vi "UIinit_setting.vi"(9 "Language":u32, 10 "VIref":refnum<vi>) -> ()   [LabVIEW 2015]
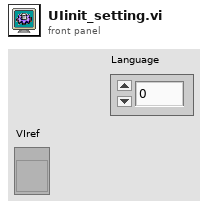
[diagram p1: front panel]
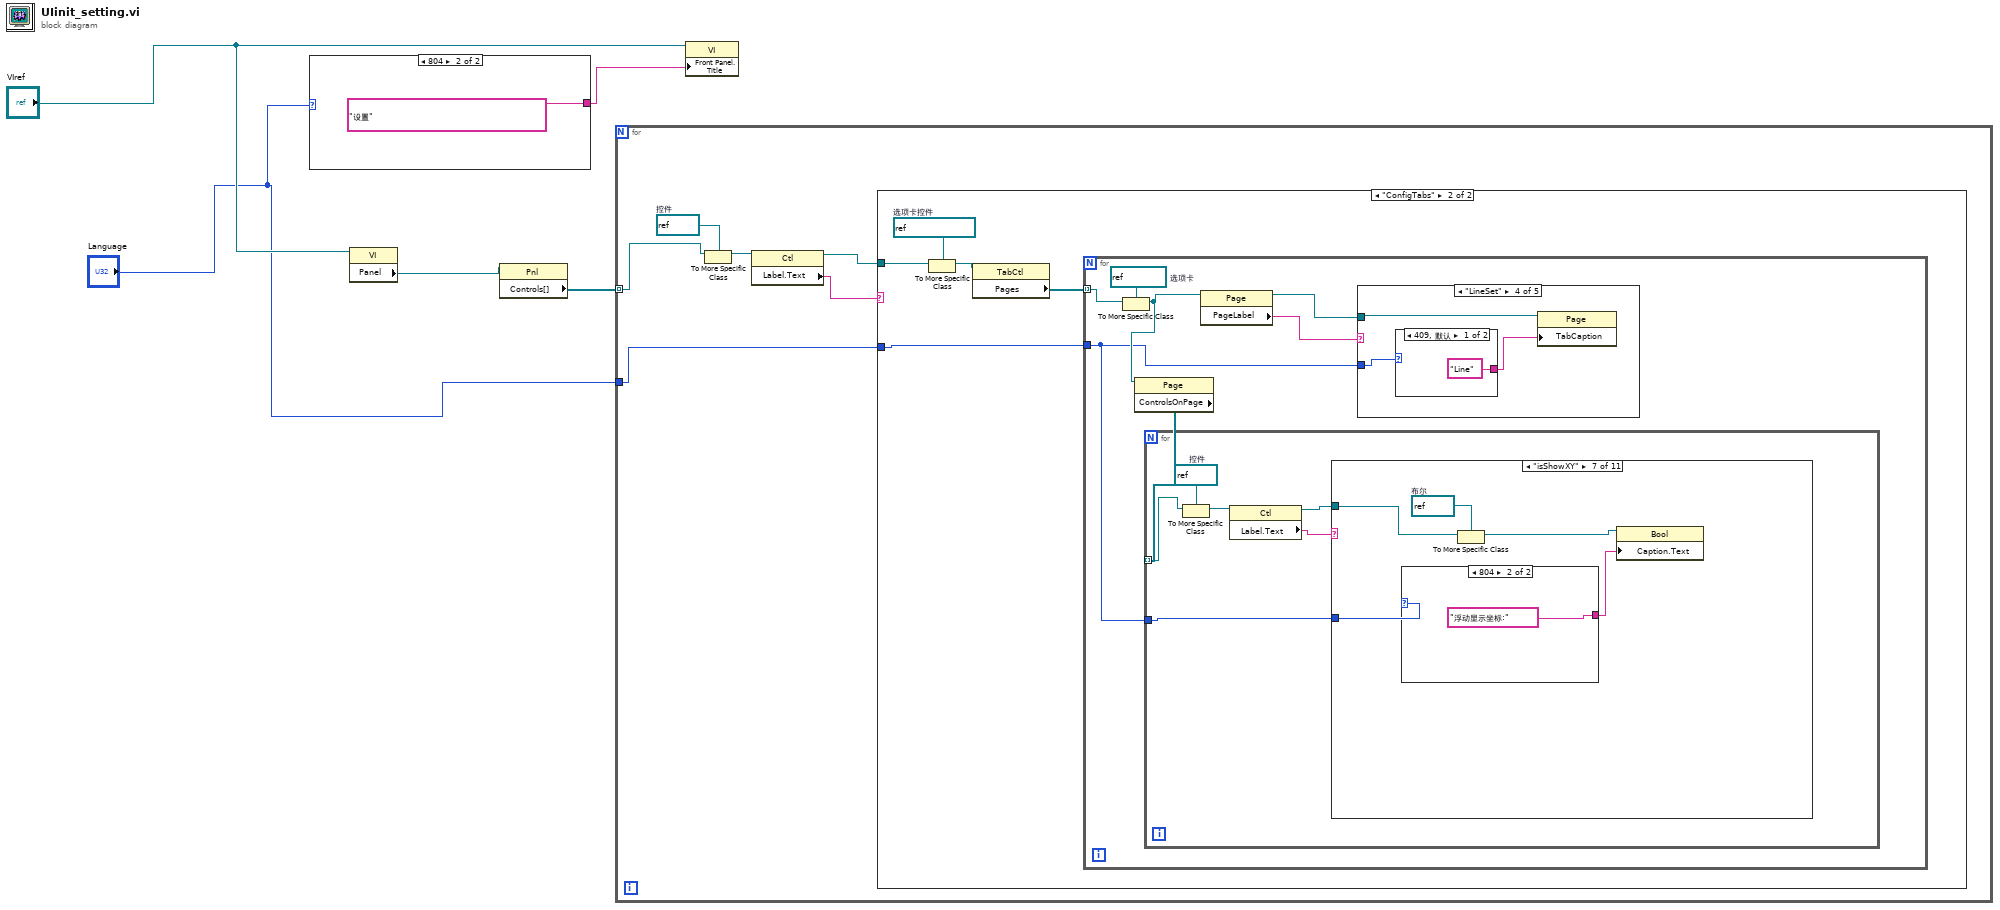
[diagram p0: block diagram]
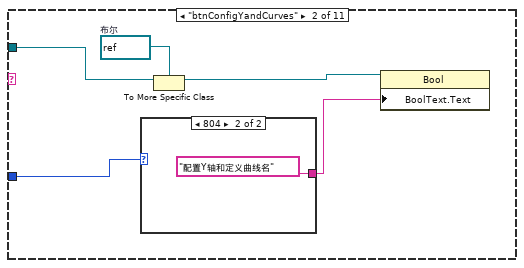
[diagram p4: hidden frame]
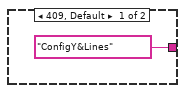
[diagram p5: hidden frame]
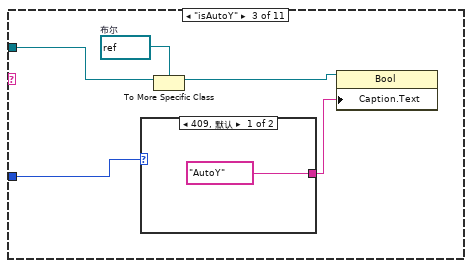
[diagram p6: hidden frame]
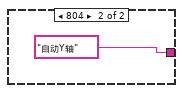
[diagram p7: hidden frame]
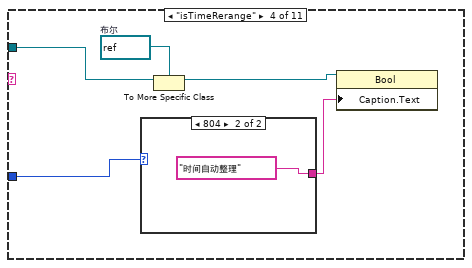
[diagram p8: hidden frame]
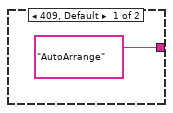
[diagram p9: hidden frame]
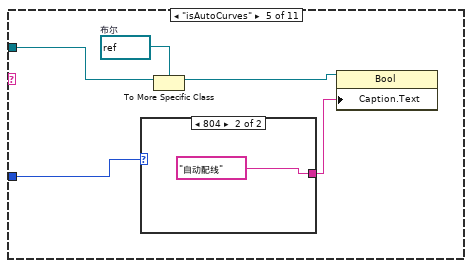
[diagram p10: hidden frame]
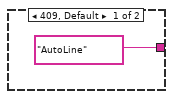
[diagram p11: hidden frame]
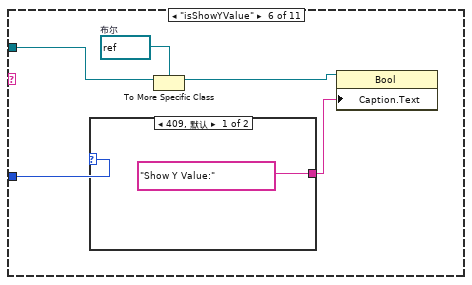
[diagram p12: hidden frame]
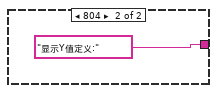
[diagram p13: hidden frame]
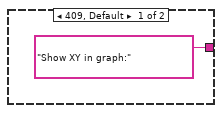
[diagram p14: hidden frame]
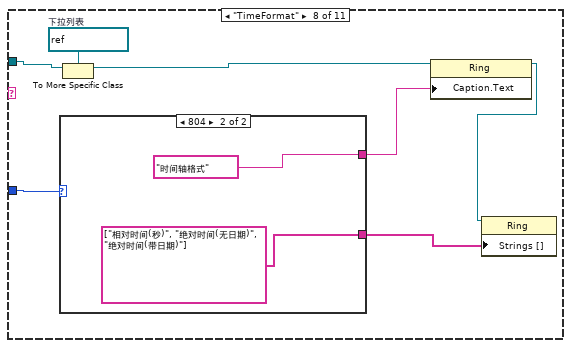
[diagram p15: hidden frame]
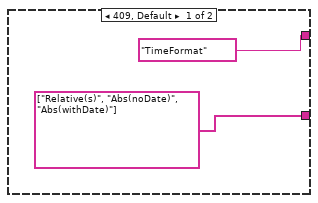
[diagram p16: hidden frame]
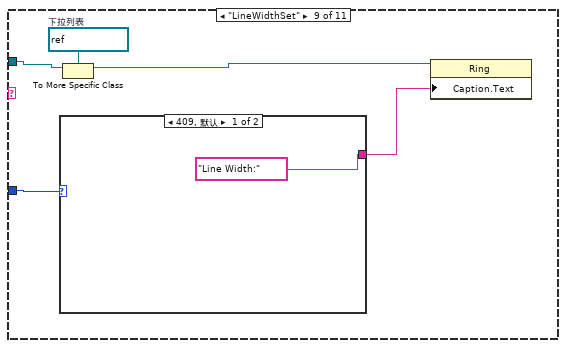
[diagram p17: hidden frame]
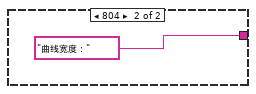
[diagram p18: hidden frame]
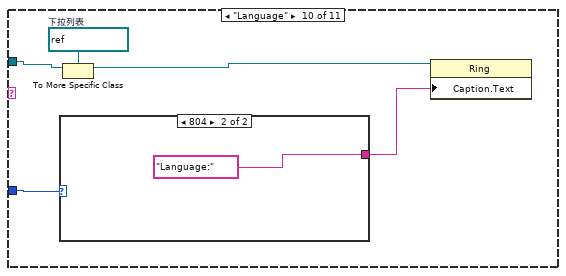
[diagram p19: hidden frame]
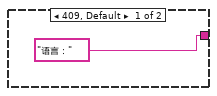
[diagram p20: hidden frame]
diagram:
  n1 = case shown="804" "Language" {
    tunnel: ["Settings" "设置"] -> w5
    frame 409, Default {
    }
    frame 804 {
    }
  }
  n2 = property class="VI"(reference="VIref") -> ("Panel"=w2:refnum<vi>)  [unwired: 1 in, 2 out]
  n3 = property class="Pnl"(reference=w2) -> ("Controls[]"=w3:refnum<vi>[])  [unwired: 1 in, 2 out]
  n4 = for {
    tunnel: w3 -> [w8] mode=indexing
    tunnel: "Language" -> [w9]
    w13 = refnum<vi> refnum  # 控件
    n5 = To More Specific Class(target class=w13, reference=w8) -> (specific class reference=w12:refnum<vi>)  [unwired: 1 in, 1 out]
    n6 = property class="Ctl"(reference=w12) -> (reference out=w10:refnum<vi>, "Label.Text"=w11:string)  [unwired: 1 in, 1 out]
    n7 = case shown="\"ConfigTabs\"" w11 {
      tunnel: w10 -> [_ w18]
      tunnel: w9 -> [_ w14]
      frame "假", Default {
      }
      frame "ConfigTabs" {
        w17 = refnum<vi> refnum  # 选项卡控件
        n8 = To More Specific Class(target class=w17, reference=w18) -> (specific class reference=w16:refnum<vi>)  [unwired: 1 in, 1 out]
        n9 = property class="TabCtl"(reference=w16) -> ("Pages"=w15:refnum<vi>[])  [unwired: 1 in, 2 out]
        n10 = for {
          tunnel: w15 -> [w22] mode=indexing
          tunnel: w14 -> [w19]
          w23 = refnum<vi> refnum  # 选项卡
          n11 = To More Specific Class(target class=w23, reference=w22) -> (specific class reference=w20:refnum<vi>)  [unwired: 1 in, 1 out]
          n12 = property class="Page"(reference=w20) -> ("ControlsOnPage"=w21:refnum<vi>[])  [unwired: 1 in, 2 out]
          n13 = for {
            tunnel: w21 -> [w26] mode=indexing
            tunnel: w19 -> [w27]
            w31 = refnum<vi> refnum  # 控件
            n14 = To More Specific Class(target class=w31, reference=w26) -> (specific class reference=w30:refnum<vi>)  [unwired: 1 in, 1 out]
            n15 = property class="Ctl"(reference=w30) -> (reference out=w28:refnum<vi>, "Label.Text"=w29:string)  [unwired: 1 in, 1 out]
            n16 = case shown="\"isShowXY\"" w29 {
              tunnel: w28 -> [_ w35 w42 w49 w56 w63 w70 w79 w88 w95 w104]
              tunnel: w27 -> [_ w36 w43 w50 w57 w64 w71 w78 w87 w94 w103]
              frame "假", Default {
              }
              frame "btnConfigYandCurves" {
                w34 = refnum<vi> refnum  # 布尔
                n17 = case shown="804" w36 {
                  tunnel: ["ConfigY&Lines" "配置Y轴和定义曲线名"] -> w32
                  frame 409, Default {
                  }
                  frame 804 {
                  }
                }
                n18 = To More Specific Class(target class=w34, reference=w35) -> (specific class reference=w33:refnum<vi>)  [unwired: 1 in, 1 out]
                n19 = property class="Bool"(reference=w33, "BoolText.Text"=w32) -> ()  [unwired: 1 in, 2 out]
              }
              frame "isAutoY" {
                w41 = refnum<vi> refnum  # 布尔
                n20 = case shown="409, 默认" w43 {
                  tunnel: ["AutoY" "自动Y轴"] -> w39
                  frame 409, Default {
                  }
                  frame 804 {
                  }
                }
                n21 = To More Specific Class(target class=w41, reference=w42) -> (specific class reference=w40:refnum<vi>)  [unwired: 1 in, 1 out]
                n22 = property class="Bool"(reference=w40, "Caption.Text"=w39) -> ()  [unwired: 1 in, 2 out]
              }
              frame "isTimeRerange" {
                w48 = refnum<vi> refnum  # 布尔
                n23 = case shown="804" w50 {
                  tunnel: ["AutoArrange" "时间自动整理"] -> w46
                  frame 409, Default {
                  }
                  frame 804 {
                  }
                }
                n24 = To More Specific Class(target class=w48, reference=w49) -> (specific class reference=w47:refnum<vi>)  [unwired: 1 in, 1 out]
                n25 = property class="Bool"(reference=w47, "Caption.Text"=w46) -> ()  [unwired: 1 in, 2 out]
              }
              frame "isAutoCurves" {
                w55 = refnum<vi> refnum  # 布尔
                n26 = case shown="804" w57 {
                  tunnel: ["AutoLine" "自动配线"] -> w53
                  frame 409, Default {
                  }
                  frame 804 {
                  }
                }
                n27 = To More Specific Class(target class=w55, reference=w56) -> (specific class reference=w54:refnum<vi>)  [unwired: 1 in, 1 out]
                n28 = property class="Bool"(reference=w54, "Caption.Text"=w53) -> ()  [unwired: 1 in, 2 out]
              }
              frame "isShowYValue" {
                w62 = refnum<vi> refnum  # 布尔
                n29 = case shown="409, 默认" w64 {
                  tunnel: ["Show Y Value:" "显示Y值定义:"] -> w60
                  frame 409, Default {
                  }
                  frame 804 {
                  }
                }
                n30 = To More Specific Class(target class=w62, reference=w63) -> (specific class reference=w61:refnum<vi>)  [unwired: 1 in, 1 out]
                n31 = property class="Bool"(reference=w61, "Caption.Text"=w60) -> ()  [unwired: 1 in, 2 out]
              }
              frame "isShowXY" {
                w69 = refnum<vi> refnum  # 布尔
                n32 = case shown="804" w71 {
                  tunnel: ["Show XY in graph:" "浮动显示坐标:"] -> w67
                  frame 409, Default {
                  }
                  frame 804 {
                  }
                }
                n33 = To More Specific Class(target class=w69, reference=w70) -> (specific class reference=w68:refnum<vi>)  [unwired: 1 in, 1 out]
                n34 = property class="Bool"(reference=w68, "Caption.Text"=w67) -> ()  [unwired: 1 in, 2 out]
              }
              frame "TimeFormat" {
                w80 = refnum<vi> refnum  # 下拉列表
                n35 = case shown="804" w78 {
                  tunnel: [string[] ["Relative(s)", "Abs(noDate)", "Abs(withDate)"] string[] ["相对时间(秒)", "绝对时间(无日期)", "绝对时间(带日期)"]] -> w77
                  tunnel: ["TimeFormat" "时间轴格式"] -> w74
                  frame 409, Default {
                  }
                  frame 804 {
                  }
                }
                n36 = To More Specific Class(target class=w80, reference=w79) -> (specific class reference=w76:refnum<vi>)  [unwired: 1 in, 1 out]
                n37 = property class="Ring"(reference=w76, "Caption.Text"=w74) -> (reference out=w75:refnum<vi>)  [unwired: 1 in, 1 out]
                n38 = property class="Ring"(reference=w75, "Strings []"=w77) -> ()  [unwired: 1 in, 2 out]
              }
              frame "LineWidthSet" {
                w89 = refnum<vi> refnum  # 下拉列表
                n39 = case shown="409, 默认" w87 {
                  tunnel: ["Line Width:" "曲线宽度："] -> w85
                  frame 409, Default {
                  }
                  frame 804 {
                  }
                }
                n40 = To More Specific Class(target class=w89, reference=w88) -> (specific class reference=w86:refnum<vi>)  [unwired: 1 in, 1 out]
                n41 = property class="Ring"(reference=w86, "Caption.Text"=w85) -> ()  [unwired: 1 in, 2 out]
              }
              frame "Language" {
                w96 = refnum<vi> refnum  # 下拉列表
                n42 = case shown="804" w94 {
                  tunnel: ["语言：" "Language:"] -> w92
                  frame 409, Default {
                  }
                  frame 804 {
                  }
                }
                n43 = To More Specific Class(target class=w96, reference=w95) -> (specific class reference=w93:refnum<vi>)  [unwired: 1 in, 1 out]
                n44 = property class="Ring"(reference=w93, "Caption.Text"=w92) -> ()  [unwired: 1 in, 2 out]
              }
              frame "ChkUpdatePeriod" {
                w105 = refnum<vi> refnum  # 下拉列表
                n45 = case shown="409, 默认" w103 {
                  tunnel: ["Check for updates:" "检查更新周期:"] -> w101
                  tunnel: [string[] ["EveryMonth", "EveryWeek", "Everyday", "EveryHour", "EveryRunning", "Never"] string[] ["每个月", "每星期", "每一天", "每小时", "每次运行", "从不"]] -> w99
                  frame 409, Default {
                  }
                  frame 804 {
                  }
                }
                n46 = To More Specific Class(target class=w105, reference=w104) -> (specific class reference=w102:refnum<vi>)  [unwired: 1 in, 1 out]
                n47 = property class="Ring"(reference=w102, "Caption.Text"=w101) -> (reference out=w100:refnum<vi>)  [unwired: 1 in, 1 out]
                n48 = property class="Ring"(reference=w100, "Strings []"=w99) -> ()  [unwired: 1 in, 2 out]
              }
            }
          }
          n49 = property class="Page"(reference=w20) -> (reference out=w24:refnum<vi>, "PageLabel"=w25:string)  [unwired: 1 in, 1 out]
          n50 = case shown="\"LineSet\"" w25 {
            tunnel: w19 -> [_ w112 w117 w122 w127]
            tunnel: w24 -> [_ w111 w116 w121 w126]
            frame "假", Default {
            }
            frame "Xset" {
              n51 = case shown="804" w112 {
                tunnel: ["X axis" "X轴"] -> w110
                frame 409, Default {
                }
                frame 804 {
                }
              }
              n52 = property class="Page"(reference=w111, "TabCaption"=w110) -> ()  [unwired: 1 in, 2 out]
            }
            frame "Yset" {
              n53 = case shown="804" w117 {
                tunnel: ["Y axis" "Y轴"] -> w115
                frame 409, Default {
                }
                frame 804 {
                }
              }
              n54 = property class="Page"(reference=w116, "TabCaption"=w115) -> ()  [unwired: 1 in, 2 out]
            }
            frame "LineSet" {
              n55 = case shown="409, 默认" w122 {
                tunnel: ["Line" "曲线"] -> w120
                frame 409, Default {
                }
                frame 804 {
                }
              }
              n56 = property class="Page"(reference=w121, "TabCaption"=w120) -> ()  [unwired: 1 in, 2 out]
            }
            frame "UI" {
              n57 = case shown="409, 默认" w127 {
                tunnel: ["Interface" "界面"] -> w125
                frame 409, Default {
                }
                frame 804 {
                }
              }
              n58 = property class="Page"(reference=w126, "TabCaption"=w125) -> ()  [unwired: 1 in, 2 out]
            }
          }
        }
      }
    }
  }
  n59 = property class="VI"(reference="VIref", "Front Panel.Title"=w5) -> ()  [unwired: 1 in, 2 out]
